vi "Robot Parameter Utility.vi"() -> ()   [LabVIEW 2015]
uses:
  Robot Parameters.ctl
  <vilib>/Utility/xml.llb/Write to XML File(string).vi
  <vilib>/Utility/xml.llb/Read From XML File(string).vi
panel:
  in  "Path":path
  in  "stop":bool
  in  "Reload":bool
  in  "Save":bool
  in  "Robot Parameters":T1
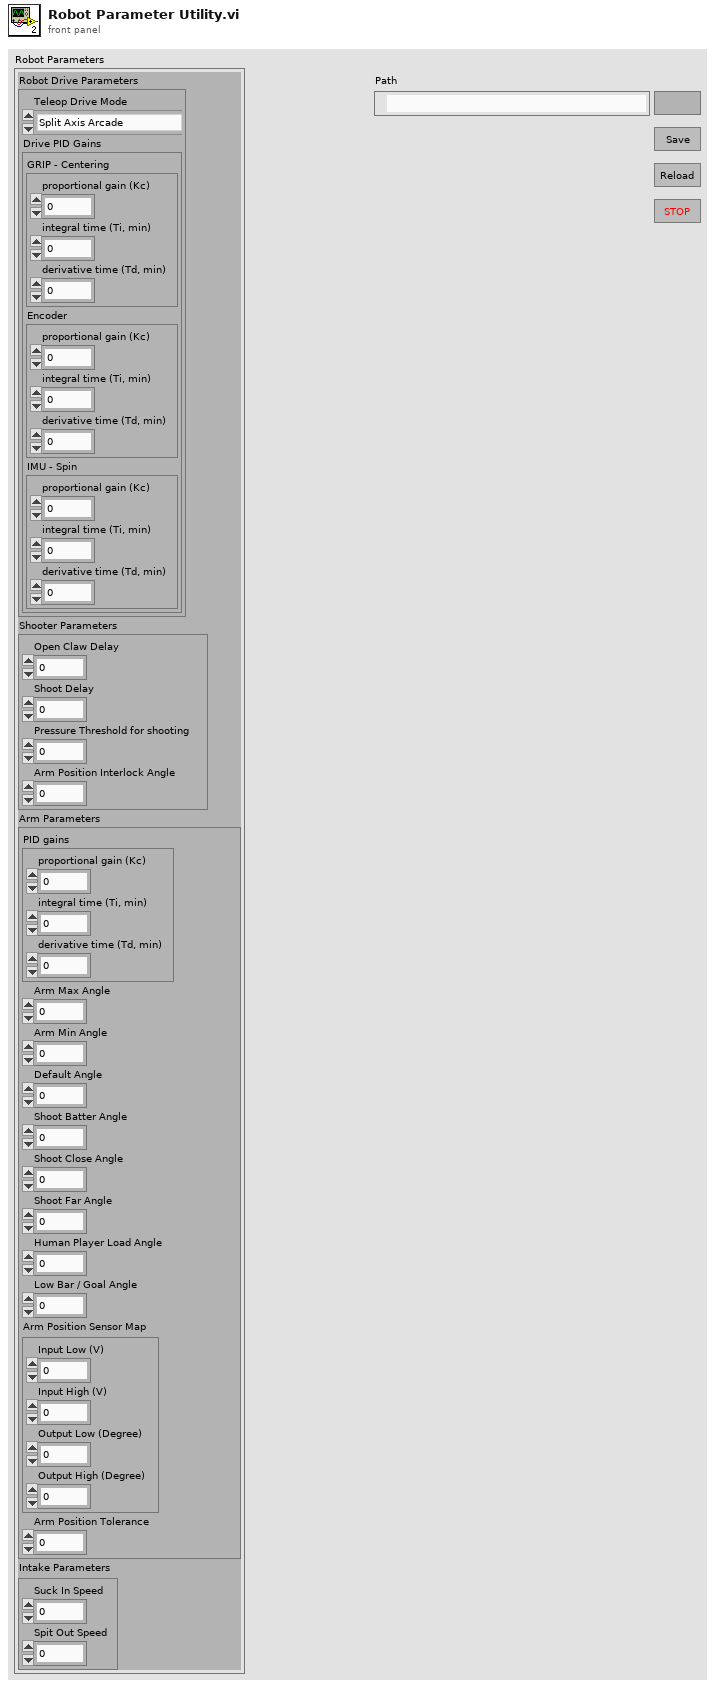
[diagram p1: front panel]
types:
  T1 = typedef "Robot Parameters.ctl" = cluster{"Robot Drive Parameters":cluster{"Teleop Drive Mode":enum16{"Split Axis Arcade", "Arcade Drive", "Tank Drive"}, "Drive PID Gains":cluster{"GRIP - Centering":cluster{"proportional gain (Kc)":dbl, "integral time (Ti, min)":dbl, "derivative time (Td, min)":dbl}, "Encoder":cluster{"proportional gain (Kc)":dbl, "integral time (Ti, min)":dbl, "derivative time (Td, min)":dbl}, "IMU - Spin":cluster{"proportional gain (Kc)":dbl, "integral time (Ti, min)":dbl, "derivative time (Td, min)":dbl}}}, "Shooter Parameters":cluster{"Open Claw Delay":u32, "Shoot Delay":u32, "Pressure Threshold for shooting":dbl, "Arm Position Interlock Angle":dbl}, "Arm Parameters":cluster{"PID gains":cluster{"proportional gain (Kc)":dbl, "integral time (Ti, min)":dbl, "derivative time (Td, min)":dbl}, "Arm Max Angle":dbl, "Arm Min Angle":dbl, "Default Angle":dbl, "Shoot Batter Angle":dbl, "Shoot Close Angle":dbl, "Shoot Far Angle":dbl, "Human Player Load Angle":dbl, "Low Bar / Goal Angle":dbl, "Arm Position Sensor Map":cluster{"Input Low (V)":dbl, "Input High (V)":dbl, "Output Low (Degree)":dbl, "Output High (Degree)":dbl}, "Arm Position Tolerance":dbl}, "Intake Parameters":cluster{"Suck In Speed":dbl, "Spit Out Speed":dbl}}
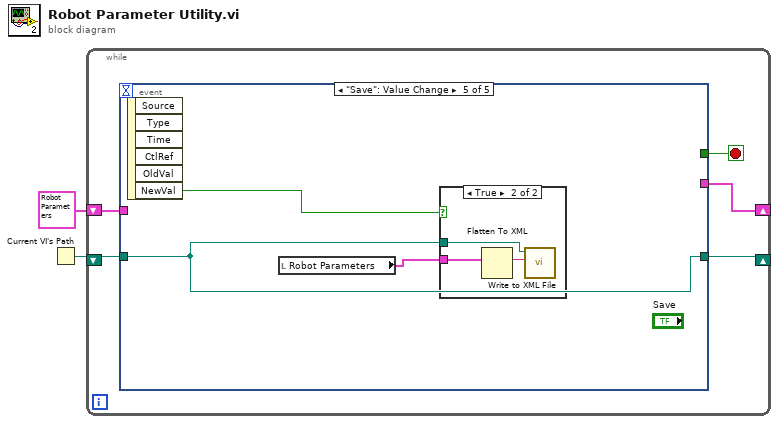
[diagram p0: block diagram]
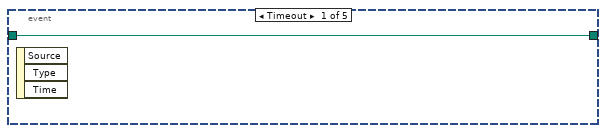
[diagram p2: hidden frame]
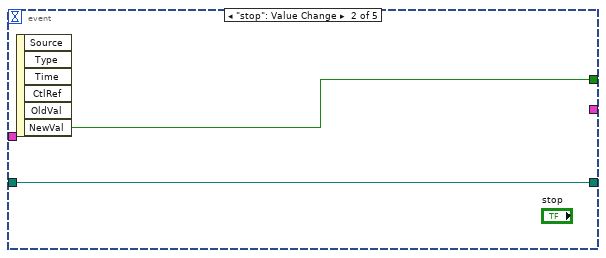
[diagram p3: hidden frame]
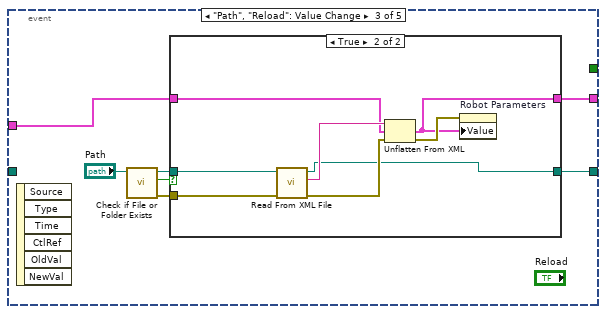
[diagram p4: hidden frame]
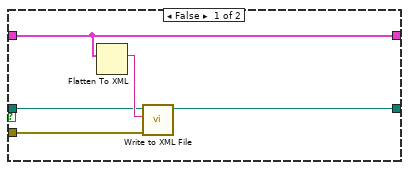
[diagram p5: hidden frame]
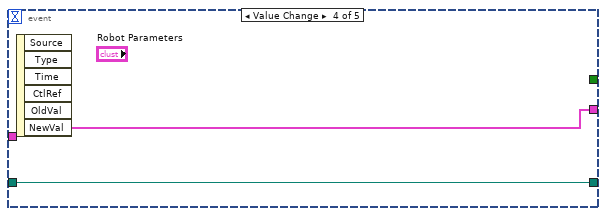
[diagram p6: hidden frame]
diagram:
  n1 = Current VI's Path() -> (path=w2:path)
  n2 = while {
    shift-right: [w6] -> _
    shift-left: w2 -> [w5]
    shift-right: [w3] -> _
    shift-left: T1 {"Robot Drive Parameters"={"Teleop Drive Mode"=enum."Split Axis Arcade", "Drive PID Gains"={"GRIP - Centering"={"proportional gain (Kc)"=0.0, "integral time (Ti, min)"=0.0, "derivative time (Td, min)"=0.0}, "Encoder"={"proportional gain (Kc)"=0.0, "integral time (Ti, min)"=0.0, "derivative time (Td, min)"=0.0}, "IMU - Spin"={"proportional gain (Kc)"=0.04000000000000001, "integral time (Ti, min)"=0.02, "derivative time (Td, min)"=0.0}}}, "Shooter Parameters"={"Open Claw Delay"=200, "Shoot Delay"=300, "Pressure Threshold for shooting"=75.0, "Arm Position Interlock Angle"=0.0}, "Arm Parameters"={"PID gains"={"proportional gain (Kc)"=0.0, "integral time (Ti, min)"=0.0, "derivative time (Td, min)"=0.0}, "Arm Max Angle"=180.0, "Arm Min Angle"=90.0, "Default Angle"=135.0, "Shoot Batter Angle"=135.0, "Shoot Close Angle"=135.0, "Shoot Far Angle"=135.0, "Human Player Load Angle"=135.0, "Low Bar / Goal Angle"=135.0, "Arm Position Sensor Map"={"Input Low (V)"=0.0, "Input High (V)"=0.0, "Output Low (Degree)"=0.0, "Output High (Degree)"=0.0}, "Arm Position Tolerance"=0.0}, "Intake Parameters"={"Suck In Speed"=0.0, "Spit Out Speed"=0.0}} ("Robot Parameters") -> [w4]
    stop <- w7 stop-if-true
    n3 = event shown="[4] \"Save\": Value Change" {
      selector: _ -> [_ _ _ _ _]
      dyn-events: _ -> [_ _ _ _ _]
      timeout: _ -> [_ _ _ _ _]
      tunnel: [_ w10 _ _ _] -> w7
      tunnel: [w8 w9 w11 w32 w34] -> w6
      tunnel: w5 -> [w8 w9 _ w32 w34]
      tunnel: w4 -> [_ _ w14 _ _]
      tunnel: [_ _ w13 w31 _] -> w3
      event Timeout {
        n4 = event-data() -> ()  [unwired: 1 in, 3 out]
      }
      event "stop": Value Change {
        n5 = event-data() -> ("NewVal"=w10:bool)  [unwired: 1 in, 5 out]
      }
      event "Path", "Reload": Value Change {
        n6 = event-data() -> ()  [unwired: 1 in, 6 out]
        n7 = call <vilib>:"Check if File or Folder Exists.vi"("path"="Path") -> ("error out"=w12:errorcluster, "file or folder exists?"=w16:bool, "dup path"=w15:path)  [unwired: 8 in]
        n8 = case shown="True" w16 {
          tunnel: w15 -> [w19 w27]
          tunnel: w14 -> [w22 w26]
          tunnel: [w22 w25] -> w13
          tunnel: w12 -> [w20 w24]
          tunnel: [w18 w23] -> w11
          frame False {
            n9 = Flatten To XML(anything=w22) -> (xml string=w21:string)
            n10 = call-poly <vilib>:"Write to XML File.vi"("error in (no error)"=w20, "XML Input"=w21, "XML File Path"=w19) -> ("XML File Path(duplicate)"=w18:path)  [unwired: 6 in, 2 out]
          }
          frame True {
            n11 = call-poly <vilib>:"Read From XML File.vi"("error in (no error)"=w24, "XML File Path"=w27) -> ("error out"=w29:errorcluster, "XML Elements"=w28:string, "XML File Path(duplicate)"=w23:path)  [unwired: 7 in]
            n12 = Unflatten From XML(xml string=w28, type=w26, error in (no error)=w29) -> (value=w25:T1, error out=w30:errorcluster)
            n13 = property on="Robot Parameters" class="Clust (strict)"(error in=w30, "Value"=w25) -> ()  [unwired: 1 in, 2 out]
          }
        }
      }
      event Value Change {
        n14 = event-data() -> ("NewVal"=w31:T1)  [unwired: 1 in, 5 out]
      }
      event "Save": Value Change {
        n15 = event-data() -> ("NewVal"=w35:bool)  [unwired: 1 in, 5 out]
        n16 = local read "Robot Parameters"() -> (w33:T1)
        n17 = case shown="True" w35 {
          tunnel: w33 -> [_ w38]
          tunnel: w34 -> [_ w36]
          frame False {
          }
          frame True {
            n18 = Flatten To XML(anything=w38) -> (xml string=w37:string)
            n19 = call-poly <vilib>:"Write to XML File.vi"("XML Input"=w37, "XML File Path"=w36) -> ()  [unwired: 7 in, 3 out]
          }
        }
      }
    }
  }
